vi "Do Updates.vi"(8 "error in (no error)":errorcluster, 11 "LightsPanel in":refnum<class "LightsPanel.lvclass">) -> (0 "error out":errorcluster, 3 "LightsPanel out":refnum<class "LightsPanel.lvclass">)   [LabVIEW 2022 SP3, in "TouchControl.lvlib" / "LightsPanel.lvclass"]
uses:
  LightsPanel.lvclass
  LightsPanel.lvclass/LightsPanel.ctl
  Update Status.ctl
  Update Type.ctl
  Light Selection.ctl
  TouchControl.lvlib
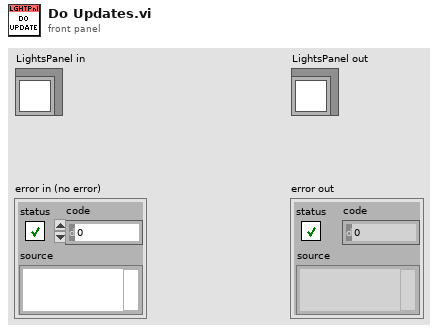
[diagram p1: front panel]
types:
  T1 = typedef "TouchControl.lvlib/Light Selection.ctl" = enum16{"Desk Left", "Desk Right", "Printer"}
  T2 = typedef "TouchControl.lvlib/LightsPanel.lvclass/Update Type.ctl" = enum16{"Light On", "Temp", "Brightness"}
  T3 = typedef "TouchControl.lvlib/LightsPanel.lvclass/Update Status.ctl" = cluster{"Set":bool, "New Value":dbl}
  T4 = typedef "TouchControl.lvlib/LightsPanel.lvclass/Update.ctl" = cluster{"Type":T2, "Light Selection":T1, "New Value":dbl}
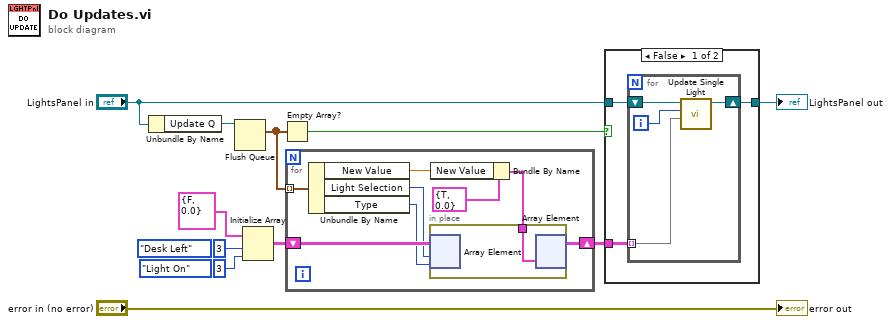
[diagram p0: block diagram]
diagram:
  (unwired) Light_Selection."Desk Left" ("Light Selection")
  (unwired) Update_Type."Light On" ("Update Type")
  n1 = Unbundle By Name("LightsPanel in") -> ("Update Q"=w6:refnum<queue>)
  n2 = Flush Queue(queue=w6) -> (remaining elements=w5:T4[])  [unwired: 1 in, 2 out]
  n3 = Initialize Array(T3 {"Set"=FALSE, "New Value"=0.0} ("Update Status"), 3 ("dimension size"), 3 ("dimension size")) -> (w7:T3[][])
  n4 = Empty Array?(array=w5) -> (empty?=w3:bool)
  n5 = for {
    shift-right: [w12] -> w1
    shift-left: w7 -> [w18]
    tunnel: w5 -> [w19] mode=indexing
    n6 = Unbundle By Name(w19) -> ("New Value"=w14:dbl, "Light Selection"=w17:T1, "Type"=w16:T2)
    n7 = Bundle By Name(cluster=T3 {"Set"=TRUE, "New Value"=0.0} ("element"), "New Value"=w14) -> (w13:T3)
    n8 = in-place {
      in-place-border: w13 -> [w20]
      n9 = in-place-array #1(w18, w17, w16) -> ()  [unwired: 1 out]
      n10 = in-place-array #1(w20) -> (w12:T3[][])  [unwired: 2 out]
    }
  }
  n11 = case shown="False" w3 {
    tunnel: "LightsPanel in" -> [w22 w28]
    tunnel: [w21 w28] -> w2
    tunnel: w1 -> [w23 _]
    frame False {
      n12 = for {
        tunnel: w23 -> [w25] mode=indexing
        shift-right: [w24] -> w21
        shift-left: w22 -> [w27]
        i -> [w26]
        n13 = call "Update Single Light.vi"("Values"=w25, "Light Selection"=w26, "LightsPanel in"=w27) -> ("LightsPanel out"=w24:refnum<class "LightsPanel.lvclass">)  [unwired: 7 in, 1 out]
      }
    }
    frame True {
      # "No updates to send"
    }
  }
  "LightsPanel out" <- w2
  "error out" <- "error in (no error)"
